vi "Konwerter UI.vi"(6 "konwersja":T1(ring), 8 "error in (no error)":errorcluster, 9 "we":dbl) -> (0 "error out":errorcluster, 1 "wy":dbl)   [LabVIEW 2019]
doc: "Converts U->I and I->U\nfor current sensors 75A, 35A 5A\nfrom series: ACS714 -5A do +5A\nand 5V supply"
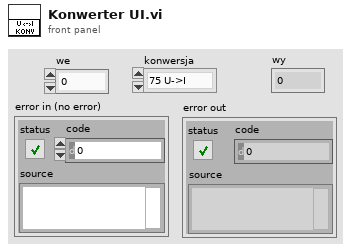
[diagram p1: front panel]
types:
  T1 = enum16{"75 U->I", "35 U->I", "5  U->I", "75  I->U", "35  I->U", "5   I->U"}
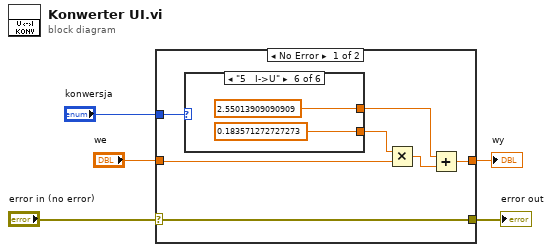
[diagram p0: block diagram]
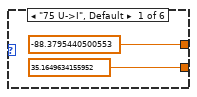
[diagram p2: hidden frame]
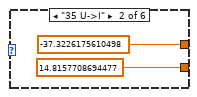
[diagram p3: hidden frame]
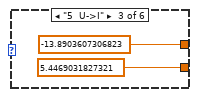
[diagram p4: hidden frame]
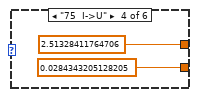
[diagram p5: hidden frame]
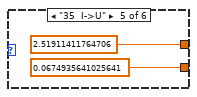
[diagram p6: hidden frame]
diagram:
  n1 = case shown="No Error" "error in (no error)" {
    selector: "error in (no error)" -> [w12 w26]
    tunnel: [w12 w26] -> w4
    tunnel: "we" -> [w10 w25]
    tunnel: [w8 w25] -> w2
    tunnel: "konwersja" -> [w11 _]
    frame No Error {
      n2 = case shown="\"5   I->U\"" w11 {
        tunnel: [35.1649634155952 14.8157708694477 5.4469031827321 0.0284343205128205 0.0674935641025641 0.183571272727273] -> w7
        tunnel: [-88.3795440500553 -37.3226175610498 -13.8903607306823 2.51328411764706 2.51911411764706 2.55013909090909] -> w6
        frame "75 U->I", Default {
        }
        frame "35 U->I" {
        }
        frame "5  U->I" {
        }
        frame "75  I->U" {
        }
        frame "35  I->U" {
        }
        frame "5   I->U" {
        }
      }
      n3 = Multiply(x=w7, y=w10) -> (x*y=w9:dbl)
      n4 = Add(x=w6, y=w9) -> (x+y=w8:dbl)
    }
    frame Error {
    }
  }
  "wy" <- w2
  "error out" <- w4
